vi "Format number_1234567890.vi"(1 "desired minimum string length":i32=10 min=1 max=10, 2 "number":i32=1445234 min=0) -> (0 "String":string)   [LabVIEW 2016]
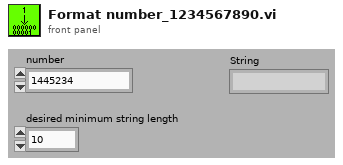
[diagram p1: front panel]
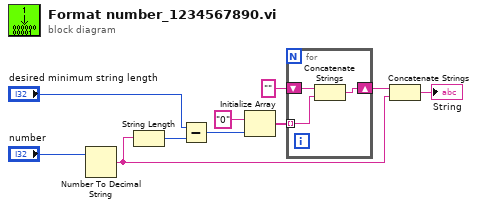
[diagram p0: block diagram]
diagram:
  n1 = Number To Decimal String(number="number") -> (decimal integer string=w9:string)  [unwired: 1 out]
  n2 = String Length(string=w9) -> (length=w4:i32)
  n3 = Subtract(x="desired minimum string length", y=w4) -> (x-y=w5:i32)
  n4 = Initialize Array("0" ("string"), w5) -> (w1:string[])
  n5 = for {
    tunnel: w1 -> [w13] mode=indexing
    shift-right: [w12] -> w6
    shift-left: "" -> [w11]
    n6 = Concatenate Strings(w11, w13) -> (w12:string)
  }
  n7 = Concatenate Strings(w6, w9) -> (→"String":string)
